vi "merFISH_initialization.vi"(7 "queue cluster":T3, 8 "Input data cluster":T1, 10 "error in":errorcluster, 11 "merFISH path":path=path "E:/") -> (1 "refnum log file":refnum<file>, 2 "Ramp":dbl[](array[numeric]), 3 "Total # z steps":i32, 4 "Ready":bool, 5 "Total # frames":i32, 6 "error out":errorcluster)   [LabVIEW 2015]
uses:
  CONTROLS/Q_FPGA_element.ctl
  CONTROLS/Q_PUMP_element.ctl
  CONTROLS/Q_VALVE_element.ctl
  CONTROLS/Q_DAQ_element.ctl
  CONTROLS/Q_camera_element.ctl
  CONTROLS/Q_ASI_stage_element.ctl
  CONTROLS/Q_MCL_piezo_element.ctl
  GLOBAL/Global_ASI_stage.vi
  GLOBAL/Global_MCL_piezo.vi
  GLOBAL/Global_DAQ.vi
  GLOBAL/Global_VALVE.vi
  GLOBAL/Global_PUMP.vi
  GLOBAL/Global_CAMERA.vi
  GLOBAL/Global_FPGA.vi
panel:
  in  "FPGA cluster":T2={"N laser lines"=0, "N Z positions"=0, "Laser lines"=[0, 0, 0, 0, 0], "Laser power"=[0.0, 0.0, 0.0, 0.0, 0.0]}
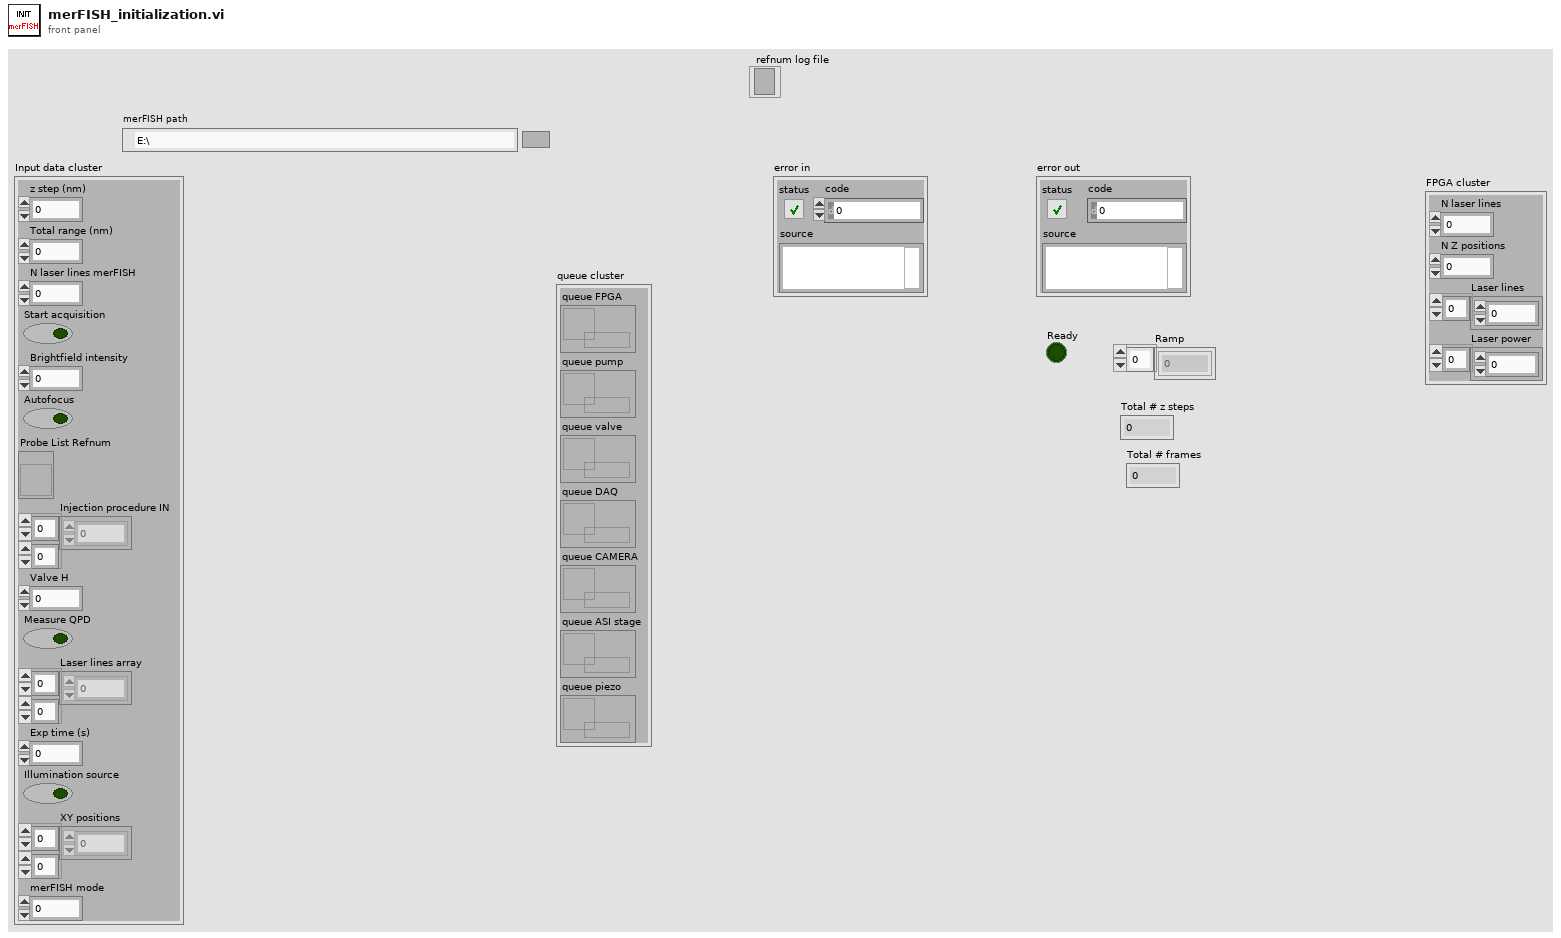
[diagram p1: front panel]
types:
  T1 = cluster{"z step (nm)":u32, "Total range (nm)":u32, "N laser lines merFISH":i32, "Start acquisition":bool, "Brightfield intensity":dbl, "Autofocus":bool, "Probe List Refnum":refnum<vi>, "Injection procedure IN":i32[][], "Valve H":u8, "Measure QPD":bool, "Laser lines array":dbl[][], "Exp time (s)":sgl, "Illumination source":bool, "XY positions":dbl[][], "merFISH mode":u16}
  T2 = cluster{"N laser lines":i32, "N Z positions":i32, "Laser lines":i32[], "Laser power":sgl[]}
  T3 = cluster{"queue FPGA":refnum<queue>, "queue pump":refnum<queue>, "queue valve":refnum<queue>, "queue DAQ":refnum<queue>, "queue CAMERA":refnum<queue>, "queue ASI stage":refnum<queue>, "queue piezo":refnum<queue>}
  T4 = typedef "Q_VALVE_element.ctl" = cluster{"variant":variant, "Instruction":enum16{"VALVE_idle", "VALVE_initialize", "VALVE_error", "VALVE_security_stop", "VALVE_change_position", "VALVE_two_way_valves", "VALVE_init_merFISH", "VALVE_stop"}}
  T5 = typedef "Q_PUMP_element.ctl" = cluster{"variant":variant, "Instruction":enum16{"PUMP_idle", "PUMP_initialize", "PUMP_error", "PUMP_security_stop", "PUMP_read_pressure", "PUMP_change_pressure", "PUMP_init_merFISH", "PUMP_change_presure_merFISH", "PUMP_zero_pressure_merFISH", "PUMP_close_merFISH", "PUMP_stop"}}
  T6 = cluster{"Total frames":i32, "Start acquisition":bool}
  T7 = typedef "Q_FPGA_element.ctl" = cluster{"variant":variant, "Instruction":enum16{"FPGA_idle", "FPGA_initialize", "FPGA_error", "FPGA_security_stop", "FPGA_laser", "FPGA_start_stop_measure_QPD", "FPGA_measure_QPD", "FPGA_measure_QPD_noise", "FPGA_stop_measure_QPD", "FPGA_init_autofocus", "FPGA_init_single_scan", "FPGA_stop_single_scan", "FPGA_init_merFISH", "FPGA_measure_QPD_merFISH", "FPGA_init_scan_merFISH", "FPGA_scan_merFISH", "FPGA_close_merFISH", "FPGA_stop"}}
  T8 = typedef "Q_ASI_stage_element.ctl" = cluster{"variant":variant, "Instruction":enum16{"ASI_idle", "ASI_initialize", "ASI_error", "ASI_security_stop", "ASI_read_XYZ", "ASI_up", "ASI_down", "ASI_left", "ASI_right", "ASI_save_XY", "ASI_move_to_XY", "ASI_brightfield", "ASI_init_scan", "ASI_init_merFISH", "ASI_move_to_XY_merFISH", "ASI_move_to_Z_merFISH", "ASI_init_autofocus_search_merFISH", "ASI_close_autofocus_search_merFISH", "ASI_adjust_piezo_autofocus_merFISH", "ASI_set_piezo_autofocus_to_reference_position_merFISH_TL", "ASI_close_merFISH", "ASI_stop"}}
  T9 = cluster{"XY ROI0":dbl[], "Brightfield intensity":dbl, "Illumination source":bool}
  T10 = typedef "Q_DAQ_element.ctl" = cluster{"variant":variant, "Instruction":enum16{"DAQ_idle", "DAQ_initialize", "DAQ_error", "DAQ_security_stop", "DAQ_init_single_scan", "DAQ_single_scan", "DAQ_init_merFISH", "DAQ_scan_merFISH", "DAQ_photobleaching_merFISH", "DAQ_close_merFISH", "DAQ_stop"}}
  T11 = typedef "Q_camera_element.ctl" = cluster{"variant":variant, "Instruction":enum16{"CAMERA_idle", "CAMERA_initialize", "CAMERA_error", "CAMERA_security_stop", "CAMERA_not_acquiring", "CAMERA_acquiring", "CAMERA_start_acquiring", "CAMERA_stop_acquiring", "CAMERA_change_exposure", "CAMERA_define_ROI", "CAMERA_cooler", "CAMERA_acquire_movie", "CAMERA_init_scan", "CAMERA_check_image_scan", "CAMERA_close_scan", "CAMERA_init_merFISH", "CAMERA_start_acquiring_merFISH", "CAMERA_close_scan_merFISH", "CAMERA_close_merFISH", "CAMERA_STOP"}}
  T12 = typedef "Q_MCL_piezo_element.ctl" = cluster{"variant":variant, "Instruction":enum16{"Piezo_idle", "Piezo_initialize", "Piezo_error", "Piezo_security_stop", "Piezo_read_z", "Piezo_move_z", "Piezo_keyboard_move", "Piezo_close_autofocus_calibration_ramp", "Piezo_change_init_state", "Piezo_init_autofocus", "Piezo_init_autofocus_merFISH_TL", "Piezo_autofocus", "Piezo_autofocus_merFISH_TL", "Piezo_stop_autofocus", "Piezo_stop_autofocus_merFISH_TL", "Piezo_autofocus_lost", "Piezo_resume_autofocus_merFISH_TL", "Piezo_check_z_position_merFISH_TL", "Piezo_init_ramp", "Piezo_move_z_ramp", "Piezo_close_ramp", "Piezo_close_merFISH", "Piezo_stop"}}
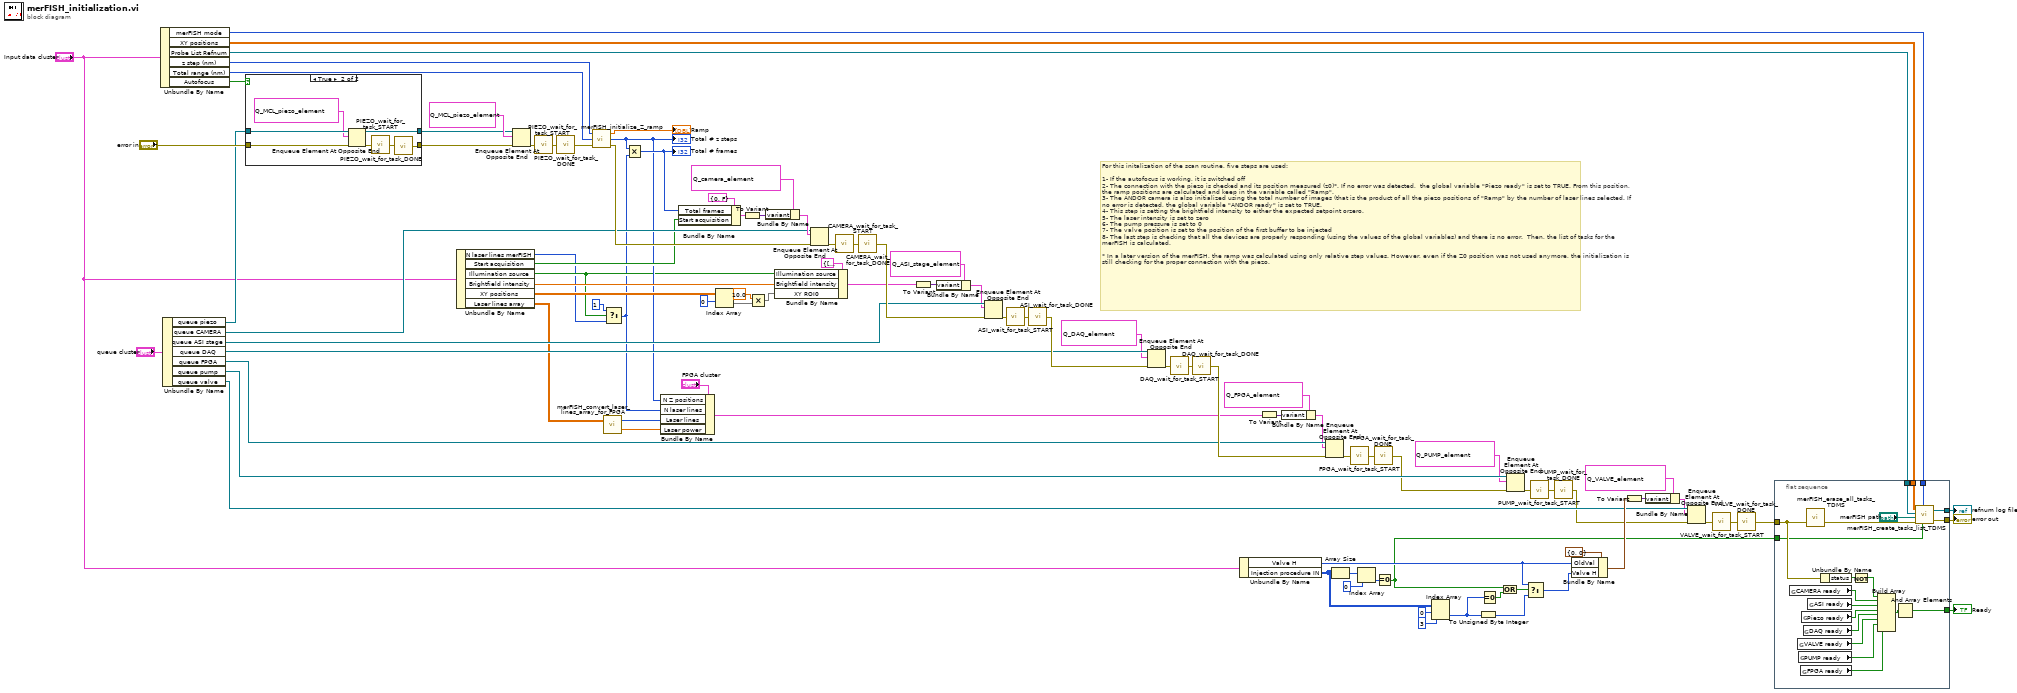
[diagram p0: block diagram]
diagram:
  # "For this initalization of the scan routine, five steps are used:\n\n1- If the autofocus is working, it is switched off\n2- The connection with the piezo is checked and its position measured (z0)*. If no error was detected,  the global variable \"Piezo ready\" is set to TRUE. From this position, the ramp positions are calculated and keep in the variable called \"Ramp\".\n3- The ANDOR camera is also initialized using the total number of images (that is the product of all the piezo positions of \"Ramp\" by the number of laser lines selected. If no error is detected, the global variable \"ANDOR ready\" is set to TRUE.\n4- This step is setting the brightfield intensity to either the expected setpoint orzero.\n5- The laser intensity is set to zero\n6- The pump pressure is set to 0\n7- The valve position is set to the position of the first buffer to be injected\n8- The last step is checking that all the devices are properly responding (using the values of the global variables) and there is no error.  Then, the list of tasks for the merFISH is calculated.\n\n* In a later version of the merFISH, the ramp was calculated using only relative step values. However, even if the Z0 position was not used anymore, the initialization is still checking for the proper connection with the piezo."
  n1 = Unbundle By Name("Input data cluster") -> ("merFISH mode"=w1:u16, "XY positions"=w13:dbl[][], "Probe List Refnum"=w41:refnum<vi>, "z step (nm)"=w73:u32, "Total range (nm)"=w72:u32, "Autofocus"=w74:bool)
  n2 = Unbundle By Name("queue cluster") -> ("queue piezo"=w78:refnum<queue>, "queue CAMERA"=w77:refnum<queue>, "queue ASI stage"=w76:refnum<queue>, "queue DAQ"=w75:refnum<queue>, "queue FPGA"=w35:refnum<queue>, "queue pump"=w37:refnum<queue>, "queue valve"=w38:refnum<queue>)
  n3 = case shown="True" w74 {
    tunnel: w78 -> [w97 w105]
    tunnel: [w97 w104] -> w80
    tunnel: "error in" -> [w98 w102]
    tunnel: [w98 w99] -> w81
    frame False {
    }
    frame True {
      n4 = Enqueue Element At Opposite End(queue=w105, element=T12 {"variant"=variant, "Instruction"=enum."Piezo_stop_autofocus"}, error in (no error)=w102) -> (queue out=w104:refnum<queue>, error out=w101:errorcluster)  [unwired: 1 in, 1 out]
      n5 = call "PIEZO_wait_for_task_START.vi"("error in"=w101) -> ("error out"=w100:errorcluster)
      n6 = call "PIEZO_wait_for_task_DONE.vi"("error in"=w100) -> ("error out"=w99:errorcluster)
    }
  }
  n7 = Unbundle By Name("Input data cluster") -> ("N laser lines merFISH"=w15:i32, "Start acquisition"=w31:bool, "Illumination source"=w16:bool, "Brightfield intensity"=w70:dbl, "XY positions"=w43:dbl[][], "Laser lines array"=w17:dbl[][])
  n8 = Enqueue Element At Opposite End(queue=w80, element=T12 {"variant"=variant, "Instruction"=enum."Piezo_init_ramp"}, error in (no error)=w81) -> (error out=w96:errorcluster)  [unwired: 1 in, 2 out]
  n9 = call "PIEZO_wait_for_task_START.vi"("error in"=w96) -> ("error out"=w95:errorcluster)
  n10 = call "PIEZO_wait_for_task_DONE.vi"("error in"=w95) -> ("error out"=w93:errorcluster)
  n11 = call "merFISH_initialize_Z_ramp.vi"("error in"=w93, "Total range (nm)"=w72, "dZ (nm)"=w73) -> ("error out"=w89:errorcluster, "Total # steps"=w24:i32, "Ramp"=→"Ramp":dbl[])
  "Total # z steps" <- w24
  n12 = call "merFISH_convert_laser_lines_array_for_FPGA.vi"("Laser lines array"=w17) -> ("Laser power"=w19:sgl[], "Laser lines"=w18:i32[])  [unwired: 1 in]
  n13 = Select(t=1, s=w16, f=w15) -> (s? t:f=w14:i32)
  n14 = Multiply(x=w24, y=w14) -> (x*y=w27:i32)
  "Total # frames" <- w27
  n15 = Bundle By Name(cluster="FPGA cluster", "N Z positions"=w24, "N laser lines"=w14, "Laser lines"=w18, "Laser power"=w19) -> (w20:T2)
  n16 = Bundle By Name(cluster=T6 {"Total frames"=0, "Start acquisition"=FALSE} ("output cluster"), "Total frames"=w27, "Start acquisition"=w31) -> (w29:T6)
  n17 = Index Array(array=w43, index (row)=0) -> (element=w45:dbl[])  [unwired: 1 in]
  n18 = To Variant(anything=w29) -> (Variant=w28:variant)
  n19 = Multiply(x=10.0, y=w45) -> (x*y=w42:dbl[])
  n20 = Bundle By Name(cluster=T11 {"variant"=variant, "Instruction"=enum."CAMERA_init_merFISH"} ("Q_ANDOR_element"), "variant"=w28) -> (w90:T11)
  n21 = Bundle By Name(cluster=T9 {"XY ROI0"=[], "Brightfield intensity"=0.0, "Illumination source"=FALSE} ("output cluster"), "Illumination source"=w16, "Brightfield intensity"=w70, "XY ROI0"=w42) -> (w69:T9)
  n22 = Enqueue Element At Opposite End(queue=w77, element=w90, error in (no error)=w89) -> (error out=w88:errorcluster)  [unwired: 1 in, 2 out]
  n23 = call "CAMERA_wait_for_task_START.vi"("error in"=w88) -> ("error out"=w87:errorcluster)
  n24 = call "CAMERA_wait_for_task_DONE.vi"("error in"=w87) -> ("error out"=w86:errorcluster)
  n25 = To Variant(anything=w69) -> (Variant=w56:variant)
  n26 = Bundle By Name(cluster=T8 {"variant"=variant, "Instruction"=enum."ASI_init_merFISH"} ("Q_ASI_stage"), "variant"=w56) -> (w55:T8)
  n27 = Enqueue Element At Opposite End(queue=w76, element=w55, error in (no error)=w86) -> (error out=w54:errorcluster)  [unwired: 1 in, 2 out]
  n28 = call "ASI_wait_for_task_START.vi"("error in"=w54) -> ("error out"=w53:errorcluster)
  n29 = call "ASI_wait_for_task_DONE.vi"("error in"=w53) -> ("error out"=w85:errorcluster)
  n30 = Enqueue Element At Opposite End(queue=w75, element=T10 {"variant"=variant, "Instruction"=enum."DAQ_init_merFISH"} ("Q_DAQ"), error in (no error)=w85) -> (error out=w40:errorcluster)  [unwired: 1 in, 2 out]
  n31 = call "DAQ_wait_for_task_START.vi"("error in"=w40) -> ("error out"=w84:errorcluster)
  n32 = call "DAQ_wait_for_task_DONE.vi"("error in"=w84) -> ("error out"=w36:errorcluster)
  n33 = Unbundle By Name("Input data cluster") -> ("Valve H"=w67:u8, "Injection procedure IN"=w66:i32[][])
  n34 = To Variant(anything=w20) -> (Variant=w21:variant)
  n35 = Bundle By Name(cluster=T7 {"variant"=variant, "Instruction"=enum."FPGA_init_merFISH"} ("element"), "variant"=w21) -> (w22:T7)
  n36 = Enqueue Element At Opposite End(queue=w35, element=w22, error in (no error)=w36) -> (error out=w34:errorcluster)  [unwired: 1 in, 2 out]
  n37 = Array Size(array=w66) -> (size(s)=w63:i32[])
  n38 = call "FPGA_wait_for_task_START.vi"("error in"=w34) -> ("error out"=w33:errorcluster)
  n39 = Index Array(array=w63, index=0) -> (element=w65:i32)
  n40 = call "FPGA_wait_for_task_DONE.vi"("error in"=w33) -> ("error out"=w32:errorcluster)
  n41 = Equal To 0?(x=w65) -> (x = 0?=w12:bool)
  n42 = Index Array(array=w66, index (row)=0, index (col)=3 ("disabled index (col)")) -> (element=w50:i32)
  n43 = To Unsigned Byte Integer(number=w50) -> (unsigned 8bit integer=w49:u8)
  n44 = Equal To 0?(x=w50) -> (x = 0?=w52:bool)
  n45 = Or(x=w12, y=w52) -> (x .or. y?=w51:bool)
  n46 = Enqueue Element At Opposite End(queue=w37, element=T5 {"variant"=variant, "Instruction"=enum."PUMP_init_merFISH"}, error in (no error)=w32) -> (error out=w10:errorcluster)  [unwired: 1 in, 2 out]
  n47 = Select(t=w67, s=w51, f=w49) -> (s? t:f=w68:u8)
  n48 = call "PUMP_wait_for_task_START.vi"("error in"=w10) -> ("error out"=w9:errorcluster)
  n49 = call "PUMP_wait_for_task_DONE.vi"("error in"=w9) -> ("error out"=w8:errorcluster)
  n50 = Bundle By Name(cluster=cluster{"Valve H":u8, "OldVal":u8} {"Valve H"=0, "OldVal"=0} ("valve positions"), "OldVal"=w67, "Valve H"=w68) -> (w59:cluster{"Valve H":u8, "OldVal":u8})
  n51 = To Variant(anything=w59) -> (Variant=w6:variant)
  n52 = Bundle By Name(cluster=T4 {"variant"=variant, "Instruction"=enum."VALVE_init_merFISH"} ("element"), "variant"=w6) -> (w5:T4)
  n53 = Enqueue Element At Opposite End(queue=w38, element=w5, error in (no error)=w8) -> (error out=w4:errorcluster)  [unwired: 1 in, 2 out]
  n54 = call "VALVE_wait_for_task_START.vi"("error in"=w4) -> ("error out"=w3:errorcluster)
  n55 = call "VALVE_wait_for_task_DONE.vi"("error in"=w3) -> ("error out"=w71:errorcluster)
  n56 = flat-sequence {
    tunnel: [w125] -> w82
    tunnel: w71 -> [w112]
    tunnel: [w114] -> w83
    tunnel: w41 -> [w109]
    tunnel: [w113] -> w58
    tunnel: w12 -> [w110]
    tunnel: w13 -> [w107]
    tunnel: w1 -> [w106]
    frame #0 {
      n57 = global read "Global_CAMERA.vi" "CAMERA ready"() -> (w122:bool)
      n58 = global read "Global_VALVE.vi" "VALVE ready"() -> (w117:bool)
      n59 = global read "Global_PUMP.vi" "PUMP ready"() -> (w116:bool)
      n60 = global read "Global_FPGA.vi" "FPGA ready"() -> (w108:bool)
      n61 = global read "Global_MCL_piezo.vi" "Piezo ready"() -> (w123:bool)
      n62 = global read "Global_DAQ.vi" "DAQ ready"() -> (w118:bool)
      n63 = call "merFISH_erase_all_tasks_TDMS.vi"("error in"=w112) -> ("error out"=w111:errorcluster)  [unwired: 2 in]
      n64 = global read "Global_ASI_stage.vi" "ASI ready"() -> (w124:bool)
      n65 = Unbundle By Name(w112) -> ("status"=w120:bool)
      n66 = Not(x=w120) -> (.not. x?=w119:bool)
      n67 = Build Array(w119, w122, w124, w123, w118, w117, w116, w108) -> (w121:bool[])
      n68 = And Array Elements(Boolean array=w121) -> (logical AND=w125:bool)
      n69 = call "merFISH_create_tasks_list_TDMS.vi"("Injection procedure empty?"=w110, "merFISH mode"=w106, "error in"=w111, "merFISH path"="merFISH path", "Probe List Refnum"=w109, "XY positions"=w107) -> ("error out"=w114:errorcluster, "refnum log file"=w113:refnum<file>)
    }
  }
  "error out" <- w83
  "Ready" <- w82
  "refnum log file" <- w58
